vi "ROS_Topic_Close_Primitive.vi"(2 "error in":errorcluster, 3 "ROS in":T1={"topic port"=0, "Node"="", "topic"="", "type"="", "node port"=0, "error "={"status"=FALSE, "code"=0, "source"=""}, "Direction"=enum."Node", "Update (ms)"=1, "queue size"=1}) -> (0 "error out":errorcluster)   [LabVIEW 2012]
doc: "Closes a topic. If no topic is defined, it will close all topics and the node."
uses:
  <userlib>/ROSforLV/ROS/Code/SubVIs/_ROSControl.ctl
  <userlib>/ROSforLV/ROS/Code/SubVIs/_ROSDirection.ctl
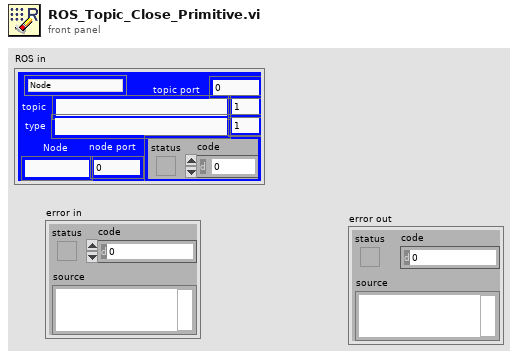
[diagram p1: front panel]
types:
  T1 = typedef "_ROSControl.ctl" = cluster{"topic port":u16, "Node":string, "topic":string, "type":string, "node port":u16, "error ":errorcluster, "Direction":T2, "Update (ms)":u16, "queue size":u16}
  T2 = typedef "_ROSDirection.ctl" = enum16{"Node", "Publisher", "Subscriber", "Service Client"}
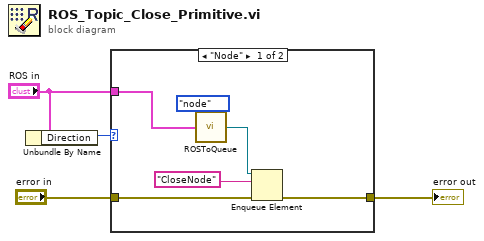
[diagram p0: block diagram]
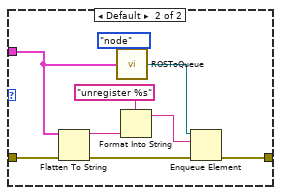
[diagram p2: hidden frame]
diagram:
  n1 = Unbundle By Name("ROS in") -> ("Direction"=w1:T2)
  n2 = case shown="\"Node\"" w1 {
    tunnel: "ROS in" -> [w7 w17]
    tunnel: "error in" -> [w6 w13]
    tunnel: [w5 w11] -> w3
    frame "Node" {
      n3 = call <userlib>:"ROSToQueue.vi"("ROS"=w7, "Name"=enum16{"topic", "node"}."node") -> ("queue"=w9:refnum<queue>)  [unwired: 2 in, 1 out]
      n4 = Enqueue Element(queue=w9, element="CloseNode" ("format string"), error in (no error)=w6) -> (error out=w5:errorcluster)  [unwired: 1 in, 2 out]
    }
    frame Default {
      n5 = Flatten To String(anything=w17, error in (no error)=w13) -> (data string=w18:string, error out=w12:errorcluster)  [unwired: 2 in, 1 out]
      n6 = call <userlib>:"ROSToQueue.vi"("ROS"=w17, "Name"=enum16{"topic", "node"}."node") -> ("queue"=w15:refnum<queue>)  [unwired: 2 in, 1 out]
      n7 = Format Into String(format string="unregister %s", w18) -> (resulting string=w14:string)  [unwired: 2 in, 1 out]
      n8 = Enqueue Element(queue=w15, element=w14, error in (no error)=w12) -> (error out=w11:errorcluster)  [unwired: 1 in, 2 out]
    }
  }
  "error out" <- w3
